vi "registerControlsEvnts.vi"(8 "error in (no error)":errorcluster, 11 "MonoPubSubData in":refnum<class "MonoPubSubData.lvclass">) -> (0 "error out":errorcluster, 2 "AllEventsRegRefnum":refnum<event-registration>, 3 "MonoPubSubData out":refnum<class "MonoPubSubData.lvclass">)   [LabVIEW 2016, in "MonoPubSubData.lvclass"]
uses:
  MonoPubSubData.lvclass
  Typedefs/slit.ctl
  Typedefs/SlitType.ctl
  Typedefs/slitWidth.ctl
  Typedefs/GratingType.ctl
  Typedefs/wavelength.ctl
  MonoPubSubData.lvclass/MonoPubSubData.ctl
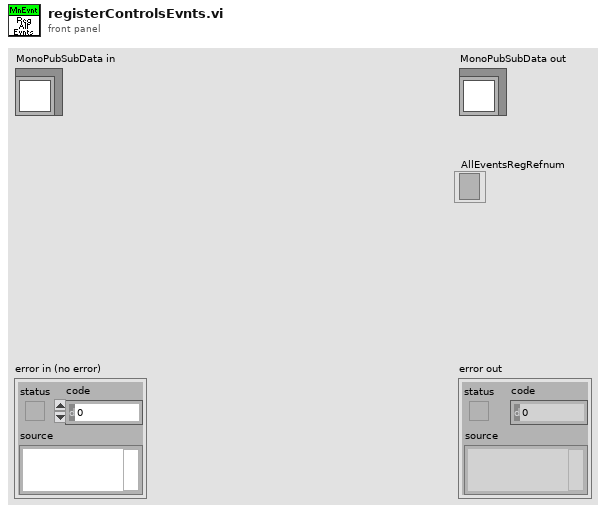
[diagram p1: front panel]
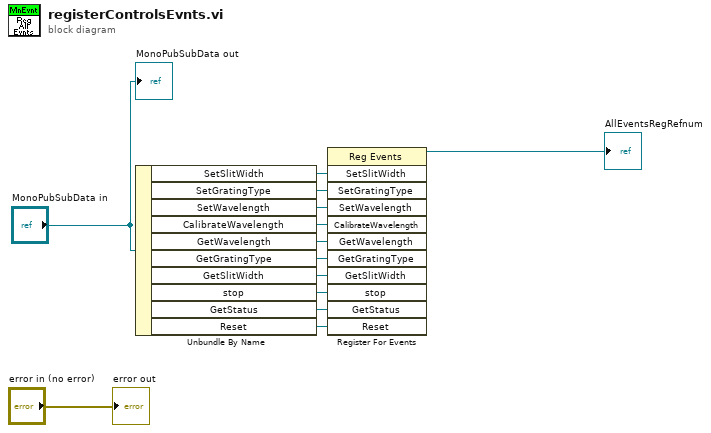
[diagram p0: block diagram]
diagram:
  n1 = Unbundle By Name("MonoPubSubData in") -> ("SetSlitWidth"=w11:refnum<user-event>, "SetGratingType"=w10:refnum<user-event>, "SetWavelength"=w9:refnum<user-event>, "CalibrateWavelength"=w8:refnum<user-event>, "GetWavelength"=w7:refnum<user-event>, "GetGratingType"=w6:refnum<user-event>, "GetSlitWidth"=w5:refnum<user-event>, "stop"=w4:refnum<user-event>, "GetStatus"=w2:refnum<user-event>, "Reset"=w1:refnum<user-event>)
  n2 = register-events(w11, w10, w9, w8, w7, w6, w5, w4, w2, w1) -> (reference out=→"AllEventsRegRefnum":refnum<event-registration>)  [unwired: 2 in, 1 out]
  "error out" <- "error in (no error)"
  "MonoPubSubData out" <- "MonoPubSubData in"
